vi "qualification round.vi"() -> ()   [LabVIEW 2018]
uses:
  <vilib>/myRIO/Instrument Drivers/Onboard IO/DIO/typedefs/DIO Reference.ctl
  <vilib>/myRIO/Common/Instrument Driver Framework/Utilities/typedefs/myRIO Generic Hardware Reference.ctl
  <vilib>/myRIO/Common/Instrument Driver Framework/Utilities/typedefs/Hardware Version Enum.ctl
  <vilib>/myRIO/Common/Instrument Driver Framework/Utilities/typedefs/myRIO v1.0 Reference.ctl
  <vilib>/myRIO/Common/Instrument Driver Framework/Utilities/typedefs/Generic FPGA Reference.ctl
  <vilib>/myRIO/Common/Instrument Driver Framework/myRIO v1.0/DIO/typedefs/DIO Channels List.ctl
  <vilib>/myRIO/Common/Instrument Driver Framework/myRIO v1.0/DIO/typedefs/DIO Channels Enum.ctl
  <vilib>/userdefined/High Color/nirio_resource_hc.ctl
  <vilib>/myRIO/Common/Instrument Driver Framework/Utilities/vis/Is FPGA Ref Available.vi
  <vilib>/myRIO/Common/Instrument Driver Framework/myRIO v1.0/DIO/vis/myRIO v1.1 Open DIO.vi
  <vilib>/myRIO/Instrument Drivers/Onboard IO/DIO/vis/Write.vi
  <vilib>/myRIO/Common/Instrument Driver Framework/Utilities/vis/Validate Channels.vi
  <vilib>/myRIO/Common/Instrument Driver Framework/myRIO v1.0/DIO/vis/myRIO v1.0 Reserve DIO.vi
  <vilib>/myRIO/Common/Instrument Driver Framework/myRIO v1.0/Resource Manager/vis/myRIO v1.0 Reserve Channel List.vi
  <vilib>/myRIO/Common/Instrument Driver Framework/myRIO v1.0/DIO/vis/myRIO v1.0 Build MUX Configuration DIO.vi
  <vilib>/myRIO/Common/Instrument Driver Framework/myRIO v1.0/Resource Manager/vis/myRIO v1.0 Reserve Channel.vi
  <vilib>/myRIO/Common/Instrument Driver Framework/myRIO v1.0/Resource Manager/vis/myRIO v1.0 Unreserve Channel.vi
  <vilib>/myRIO/Common/Instrument Driver Framework/myRIO v1.0/Resource Manager/vis/myRIO v1.0 Create Configuration List.vi
  <vilib>/myRIO/Common/Instrument Driver Framework/myRIO v1.0/Resource Manager/vis/myRIO v1.0 Build Mutex Name.vi
  vision/vision info 2.vi
  <vilib>/Utility/VariantDataType/GetNumericInfo.vi
  <vilib>/Utility/error.llb/Error Cluster From Error Code.vi
  <vilib>/myRIO/Common/Instrument Driver Framework/myRIO v1.0/myRIO v1.1 Open.vi
  <vilib>/myRIO/Common/Instrument Driver Framework/Utilities/vis/IO Manager.vi
  <vilib>/myRIO/Common/Instrument Driver Framework/Utilities/vis/Configuration Manager.vi
  <vilib>/myRIO/Common/Instrument Driver Framework/myRIO v1.0/Resource Manager/vis/myRIO v1.0 Configure IO.vi
  <vilib>/myRIO/Common/Instrument Driver Framework/myRIO v1.0/myRIO v1.0 Close.vi
  <vilib>/myRIO/Common/Instrument Driver Framework/myRIO v1.0/DIO/vis/myRIO v1.0 Write DIO.vi
  <vilib>/myRIO/Express VI/Onboard Devices/LED/LED Express VI.xnode
  <vilib>/myRIO/Instrument Drivers/Onboard IO/DIO/vis/myRIO DIO Open.xnode
  <vilib>/myRIO/Instrument Drivers/Onboard IO/DIO/DIO.lvlib
  <vilib>/myRIO/Instrument Drivers/Onboard IO/DIO/vis/Read.vi
  <vilib>/myRIO/Express VI/Onboard Devices/Button/Button Express VI.xnode
  <vilib>/myRIO/Express VI/Onboard IO/DI/DI Express VI.xnode
panel:
  out "stack cube":enum16{"Z", "I", "O", "S", "L", "J", "T", "N"}(ring)
  out "Value":bool
  out "Boolean":bool
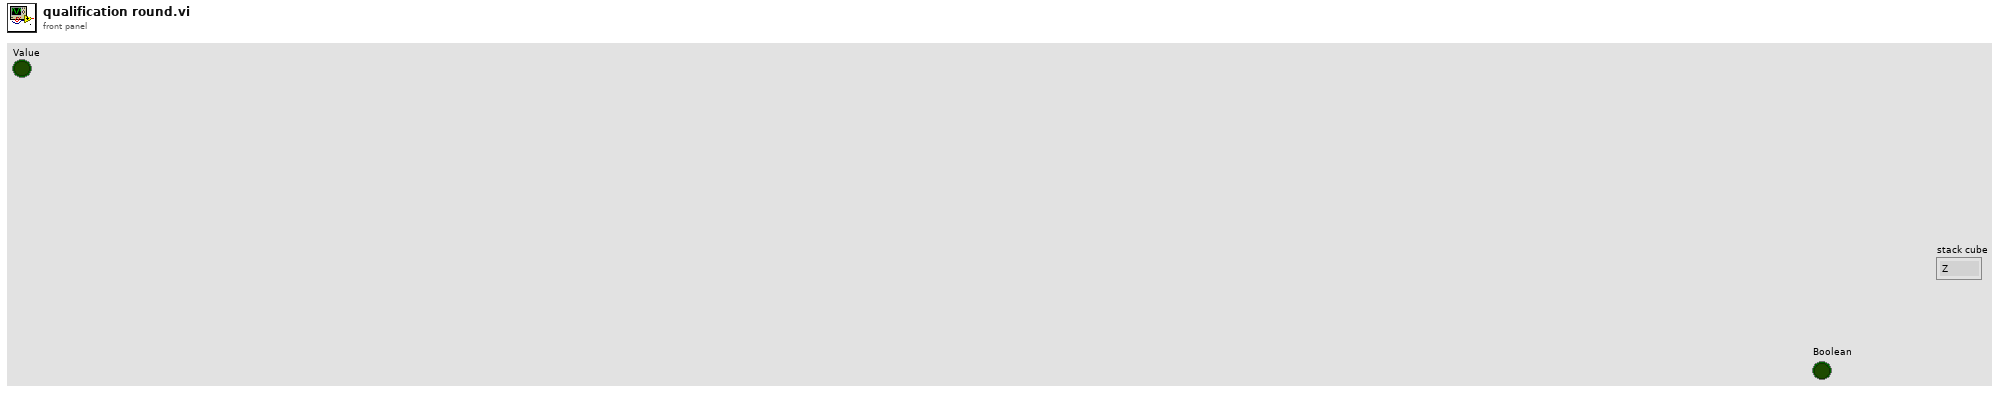
[diagram p1: front panel]
types:
  T1 = typedef "DIO.lvlib/DIO Reference.ctl" = cluster{"myRIO Reference":T2, "DIO Channels List":T6}
  T2 = typedef "myRIO Generic Hardware Reference.ctl" = cluster{"myRIO Model":T3, "myRIO Hardware Reference":T4}
  T3 = typedef "Hardware Version Enum.ctl" = enum16{"Unknown", "myRIO-1900", "myRIO-1950", "roboRIO", "NI ELVIS RIO CM", "ELVIS III"}
  T4 = typedef "myRIO v1.0 Reference.ctl" = cluster{"Generic FPGA Reference":T5, "Allow multiple opens":bool}
  T5 = typedef "Generic FPGA Reference.ctl" = refnum<k20>
  T6 = typedef "DIO Channels List.ctl" = T7[]
  T7 = typedef "DIO Channels Enum.ctl" = enum16{"Not Connected", "C/DIO0", "C/DIO1", "C/DIO2", "C/DIO3", "C/DIO4", "C/DIO5", "C/DIO6", "C/DIO7", "A/DIO0", "A/DIO1", "A/DIO2", "A/DIO3", "A/DIO4", "A/DIO5", "A/DIO6", "A/DIO7", "A/DIO8", "A/DIO9", "A/DIO10", "A/DIO11", "A/DIO12", "A/DIO13", "A/DIO14", "A/DIO15", "A/DIO16", "A/DIO17", "A/DIO18", "A/DIO19", "B/DIO0", "B/DIO1", "B/DIO2", "B/DIO3", "B/DIO4", "B/DIO5", "B/DIO6", "B/DIO7", "B/DIO8", "B/DIO9", "B/DIO10", "B/DIO11", "B/DIO12", "B/DIO13", "B/DIO14", "B/DIO15", "B/DIO16", "B/DIO17", "B/DIO18", "B/DIO19", "LED0", "LED1", "LED2", "LED3", "Button0", "DIO/DIO0", "DIO/DIO1", "DIO/DIO2", "DIO/DIO3", "DIO/DIO4", "DIO/DIO5", "DIO/DIO6", "DIO/DIO7", "DIO/DIO8", "DIO/DIO9", "SPI/CS0", "SPI/CS1", "SPI/CS2", "SPI/CS3", "LED RADIO (Green)", "LED RADIO (Red)", "LED COMM (Green)", "LED COMM (Red)", "LED MODE (Green)", "LED MODE (Red)"}
  T8 = typedef "nirio_resource_hc.ctl" = tag
  T9 = enum16{"shoulder", "elbow", "wrist", "base", "gripper"}
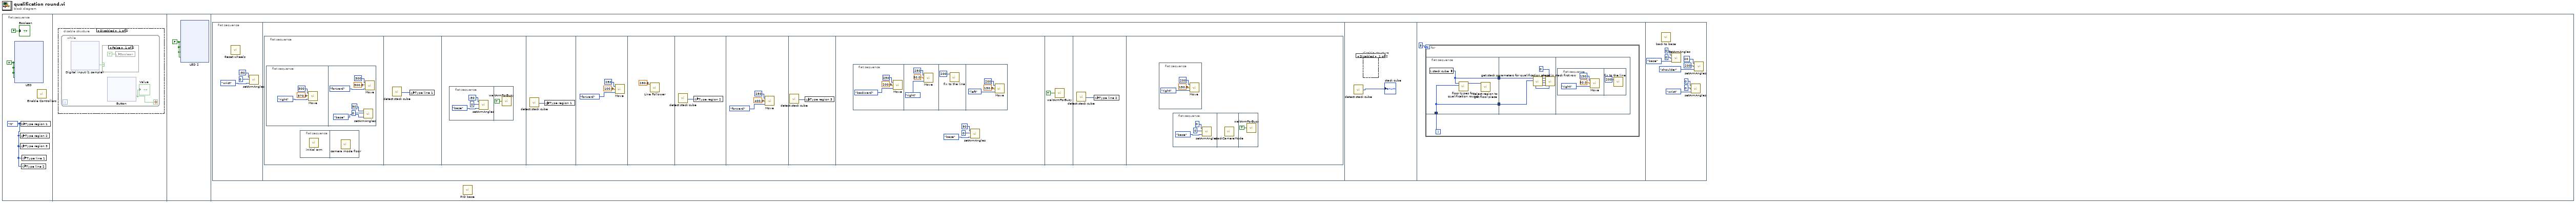
[diagram p0: block diagram]
diagram:
  n1 = flat-sequence {
    frame #0 {
      w1 = enum16{"Z", "I", "O", "S", "L", "J", "T", "N"}."N" ("Type region 1")
      w3 = TRUE ("LED0")
      n2 = xnode "LED"("LED0"=w3, "LED1"=w3, "LED2"=w3, "LED3"=w3) -> ()  [unwired: 1 in, 1 out]
      n3 = global write "vision info 2.vi" "Type region 2"(w1) -> ()
      n4 = global write "vision info 2.vi" "Type region 3"(w1) -> ()
      n5 = global write "vision info 2.vi" "Type region 1"(w1) -> ()
      n6 = global write "vision info 2.vi" "Type line 2"(w1) -> ()
      n7 = global write "vision info 2.vi" "Type line 1"(w1) -> ()
      n8 = call "Enable Controllers.vi"() -> ()  [unwired: 12 in]
      "Boolean" <- FALSE ("Boolean")
    }
    frame #1 {
      n9 = disable-structure shown="Disabled" {
        frame Disabled {
          n10 = while {
            stop <- w43 stop-if-true
            n11 = xnode "Digital input (1 sample)"() -> ("A/DIO0 (Pin 11)"=w42:bool)  [unwired: 1 in, 1 out]
            n12 = case shown="False" w42 {
              frame False {
                n13 = local write "Boolean"(TRUE ("Boolean")) -> ()
              }
              frame True {
              }
            }
            n14 = xnode "Button"() -> ("Value"=w43:bool)  [unwired: 1 in, 1 out]
            "Value" <- w43
          }
        }
        frame Enabled {
        }
      }
    }
    frame #2 {
      w115 = FALSE ("LED0")
      n15 = xnode "LED 2"("LED0"=w115, "LED1"=w115, "LED2"=w115, "LED3"=w115) -> ()  [unwired: 1 in, 1 out]
    }
    frame #3 {
      n16 = flat-sequence {
        frame #0 {
          n17 = call "Reset wheels.vi"() -> ()  [unwired: 12 in]
          n18 = call "setArmAngles.vi"("Enum"=T9."wrist", "speed"=0, "angle"=-90) -> ()  [unwired: 1 in]
        }
        frame #1 {
          n19 = flat-sequence {
            frame #0 {
              n20 = flat-sequence {
                frame #0 {
                  n21 = call "Move.vi"("Enum"=enum16{"forward", "backward", "left", "right"}."right", "distance"=570.0, "speed"=300) -> ()  [unwired: 1 in]
                }
                frame #1 {
                  n22 = call "setArmAngles.vi"("Enum"=T9."base", "speed"=0, "angle"=90) -> ()  [unwired: 1 in]
                  n23 = call "Move.vi"("Enum"=enum16{"forward", "backward", "left", "right"}."forward", "distance"=500.0, "speed"=300) -> ()  [unwired: 1 in]
                }
              }
              n24 = flat-sequence {
                frame #0 {
                  n25 = call "initial arm.vi"() -> ()  [unwired: 12 in]
                }
                frame #1 {
                  n26 = call "camera mode floor.vi"() -> ()  [unwired: 12 in]
                }
              }
            }
            frame #1 {
              n27 = call "detect stack cube.vi"() -> ("Type"=w166:enum16{"Z", "I", "O", "S", "L", "J", "T", "N"})
              n28 = global write "vision info 2.vi" "Type line 1"(w166) -> ()
            }
            frame #2 {
              n29 = flat-sequence {
                frame #0 {
                  n30 = call "setArmAngles.vi"("Enum"=T9."base", "speed"=0, "angle"=-90) -> ()  [unwired: 1 in]
                }
                frame #1 {
                  n31 = call "waitArmForBusy.vi"("base"=TRUE) -> ()
                }
              }
            }
            frame #3 {
              n32 = call "detect stack cube.vi"() -> ("Type"=w171:enum16{"Z", "I", "O", "S", "L", "J", "T", "N"})
              n33 = global write "vision info 2.vi" "Type region 1"(w171) -> ()
            }
            frame #4 {
              n34 = call "Move.vi"("Enum"=enum16{"forward", "backward", "left", "right"}."forward", "distance"=100.0, "speed"=250) -> ()  [unwired: 1 in]
            }
            frame #5 {
              n35 = call "Line Follower.vi"("speed"=280.0) -> ()  [unwired: 11 in]
            }
            frame #6 {
              n36 = call "detect stack cube.vi"() -> ("Type"=w176:enum16{"Z", "I", "O", "S", "L", "J", "T", "N"})
              n37 = global write "vision info 2.vi" "Type region 2"(w176) -> ()
            }
            frame #7 {
              n38 = call "Move.vi"("Enum"=enum16{"forward", "backward", "left", "right"}."forward", "distance"=400.0, "speed"=250) -> ()  [unwired: 1 in]
            }
            frame #8 {
              n39 = call "detect stack cube.vi"() -> ("Type"=w180:enum16{"Z", "I", "O", "S", "L", "J", "T", "N"})
              n40 = global write "vision info 2.vi" "Type region 3"(w180) -> ()
            }
            frame #9 {
              n41 = flat-sequence {
                frame #0 {
                  n42 = call "Move.vi"("Enum"=enum16{"forward", "backward", "left", "right"}."backward", "distance"=200.0, "speed"=250) -> ()  [unwired: 1 in]
                }
                frame #1 {
                  n43 = call "Move.vi"("Enum"=enum16{"forward", "backward", "left", "right"}."right", "distance"=50.0, "speed"=250) -> ()  [unwired: 1 in]
                }
                frame #2 {
                  n44 = call "fix to the line.vi"("speed"=200) -> ()  [unwired: 11 in]
                }
                frame #3 {
                  n45 = call "Move.vi"("Enum"=enum16{"forward", "backward", "left", "right"}."left", "distance"=150.0, "speed"=200) -> ()  [unwired: 1 in]
                }
              }
              n46 = call "setArmAngles.vi"("Enum"=T9."base", "speed"=0, "angle"=90) -> ()  [unwired: 1 in]
            }
            frame #10 {
              n47 = call "waitArmForBusy.vi"("base"=TRUE) -> ()
            }
            frame #11 {
              n48 = call "detect stack cube.vi"() -> ("Type"=w195:enum16{"Z", "I", "O", "S", "L", "J", "T", "N"})
              n49 = global write "vision info 2.vi" "Type line 2"(w195) -> ()
            }
            frame #12 {
              n50 = flat-sequence {
                frame #0 {
                  n51 = call "Move.vi"("Enum"=enum16{"forward", "backward", "left", "right"}."right", "distance"=150.0, "speed"=200) -> ()  [unwired: 1 in]
                }
              }
              n52 = flat-sequence {
                frame #0 {
                  n53 = call "setArmAngles.vi"("Enum"=T9."base", "speed"=0, "angle"=0) -> ()  [unwired: 1 in]
                }
                frame #1 {
                  n54 = call "stackCameraMode.vi"() -> ()  [unwired: 12 in]
                }
                frame #2 {
                  n55 = call "waitArmForBusy.vi"("base"=TRUE) -> ()
                }
              }
            }
          }
        }
        frame #2 {
          n56 = call "detect stack cube.vi"() -> ("Type"=→"stack cube":enum16{"Z", "I", "O", "S", "L", "J", "T", "N"})
          n57 = disable-structure shown="Disabled" {
            frame Disabled {
            }
            frame Enabled {
            }
          }
        }
        frame #3 {
          n58 = for {
            N: 5 -> [_]
            i -> [w206]
            n59 = flat-sequence {
              tunnel: w206 -> [w208]
              tunnel: [w209] -> w207
              tunnel: [w208] -> w205
              tunnel: w207 -> [w213]
              tunnel: w205 -> [w211]
              frame #0 {
                n60 = local read "stack cube"() -> (w209:enum16{"Z", "I", "O", "S", "L", "J", "T", "N"})
                n61 = call "floor types for qualification round.vi"("cnt"=w208, "Type"=w209) -> ("Type required"=w210:enum16{"Z", "I", "O", "S", "L", "J", "T", "N"})  [unwired: 9 in]
                n62 = call "select region to get floor piece.vi"("type"=w210) -> ()  [unwired: 11 in]
              }
              frame #1 {
                n63 = call "get stack parameters for qualification round.vi"("cnt"=w211, "Type"=w213) -> ("ang2"=w215:i8, "ang1"=w216:i8, "c2"=w217:i16, "c1"=w218:i16, "row"=w212:i8)  [unwired: 1 in]
                n64 = call "place in stack first row.vi"("row"=w212, "base ang"=0, "angle 2"=w215, "angle"=w216, "c2"=w217, "c1"=w218) -> ()  [unwired: 6 in]
              }
              frame #2 {
                n65 = flat-sequence {
                  frame #0 {
                    n66 = call "Move.vi"("Enum"=enum16{"forward", "backward", "left", "right"}."right", "distance"=50.0, "speed"=130) -> ()  [unwired: 1 in]
                  }
                  frame #1 {
                    n67 = call "fix to the line.vi"("speed"=200) -> ()  [unwired: 11 in]
                  }
                }
              }
            }
          }
        }
        frame #4 {
          n68 = call "back to base.vi"() -> ()  [unwired: 12 in]
          n69 = call "setArmAngles.vi"("Enum"=T9."base", "speed"=0, "angle"=0) -> ()  [unwired: 1 in]
          n70 = call "setArmAngles.vi"("Enum"=T9."wrist", "speed"=0, "angle"=0) -> ()  [unwired: 1 in]
          n71 = call "setArmAngles.vi"("Enum"=T9."shoulder", "speed"=200, "angle"=20) -> ()  [unwired: 1 in]
        }
      }
      n72 = call "PID base.vi"() -> ()  [unwired: 12 in]
    }
  }
